vi "_Table Test.vi"   [LabVIEW 2015]
uses:
  <vilib>/rvi/Emulation/niFpgaSctlEmulationResourceMgr.vi
  <vilib>/rvi/Memory/Memory_Emulation/nirvimemoryEmulationManagerCache_SetValue.vi
  <vilib>/rvi/Emulation/niFpgaSctlEmulationGetInTimedLoop.vi
  <vilib>/rvi/Emulation/niFpgaEmulationIsFPGAContextNoSignature.vi
  <vilib>/rvi/Memory/Memory_Emulation/nirvimemoryEmulationManagerCache_GetValue.vi
  <vilib>/rvi/Memory/Memory_Emulation/nirvimemoryEmulationManagerCache_ReleaseExclusive.vi
  <vilib>/Utility/error.llb/Clear Errors.vi
  <vilib>/rvi/Memory/Memory_Emulation/nirvimemoryEmulationManagerCache_InsertValue.vi
  <vilib>/rvi/Memory/Memory_Emulation/niFpgaMemoryEmulationValidateCache.vi
  <vilib>/rvi/Memory/Memory_Emulation/nirvimemoryEmulationManagerCache_MakeExclusive.vi
  <vilib>/rvi/Memory/Memory_Emulation/niFpgaMemoryEmulationCacheClearOnFirstRun.vi
  <vilib>/rvi/DataTransferAndStorage/Container/Common/niFpgaContainerGetUniqueNameForEmu.vi
  <vilib>/rvi/Memory/Memory_Emulation/nirvimemoryEmulation.vi
  <vilib>/rvi/Memory/Memory_Emulation/nirvimemoryFastEmulation.vi
  <vilib>/rvi/DataTransferAndStorage/Container/XNode/niFpgaContainer.xnode
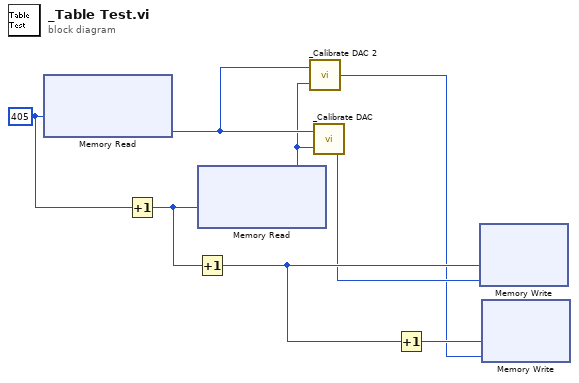
[diagram p0: block diagram]
diagram:
  w8 = u32 405 ("Address")
  n1 = xnode "Memory Read"("Address"=w8) -> ("Data"=w7:u32)  [unwired: 1 in, 1 out]
  n2 = Increment(x=w8) -> (x+1=w5:u32)
  n3 = Increment(x=w5) -> (x+1=w4:u32)
  n4 = xnode "Memory Read"("Address"=w5) -> ("Data"=w6:u32)  [unwired: 1 in, 1 out]
  n5 = call "_Calibrate DAC 2.vi"("Table Type"=w6, "Current Mass"=w7) -> ("DAC"=w1:u32)
  n6 = call "_Calibrate DAC.vi"("Table Type"=w6, "Current Mass"=w7) -> ("DAC"=w2:u32)
  n7 = Increment(x=w4) -> (x+1=w3:u32)
  n8 = xnode ("Memory Write")("Address"=w4, "Data"=w2) -> ()  [unwired: 1 in, 1 out]
  n9 = xnode ("Memory Write")("Address"=w3, "Data"=w1) -> ()  [unwired: 1 in, 1 out]
